vi "reponsegetport.vi"(8 "error in (no error)":errorcluster, 11 "simulado in":refnum<class "simulado.lvclass">) -> (0 "error out":errorcluster, 2 "String":string, 3 "simulado out":refnum<class "simulado.lvclass">)   [LabVIEW 2019, in "simulado.lvclass"]
uses:
  simulado.lvclass
  simulado.lvclass/simulado.ctl
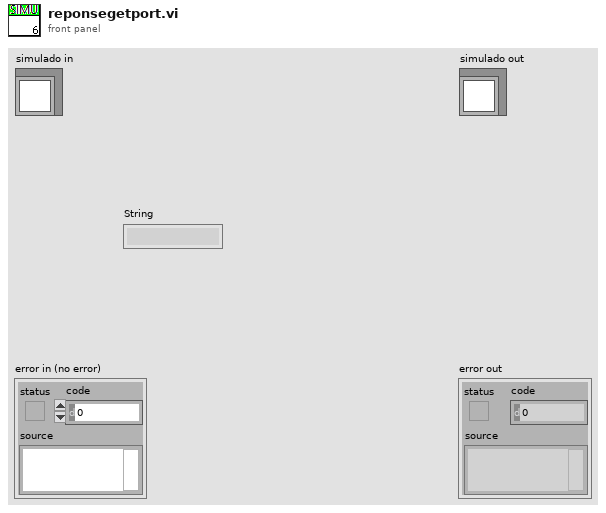
[diagram p1: front panel]
types:
  T1 = enum16{"get parameter", "Set parameters", "reset parameter", ""}
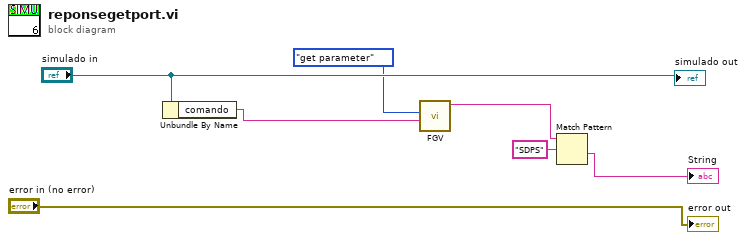
[diagram p0: block diagram]
diagram:
  n1 = Unbundle By Name("simulado in") -> ("comando"=w6:string)
  n2 = call "FGV.vi"("command"=w6, "functions"=T1."get parameter") -> ("response retrirvrd"=w4:string)  [unwired: 8 in, 1 out]
  n3 = Match Pattern(string=w4, regular expression="SDPS") -> (after substring=→"String":string)  [unwired: 1 in, 3 out]
  "error out" <- "error in (no error)"
  "simulado out" <- "simulado in"
